vi "Lab13_ThingWorx_WriteToCloud_Bennett.vi"() -> ()   [LabVIEW 2016]
uses:
  <vilib>/National Instruments/IoT Education Toolkit Beta/TW API/TW_SetPropertyValue_Int_Public.vi
  <vilib>/National Instruments/IoT Education Toolkit Beta/TW API/TW_SetPropertyValue_Timestamp_Public.vi
  <vilib>/National Instruments/IoT Education Toolkit Beta/TW API/TW_SetPropertyValue_String_Public.vi
  <vilib>/National Instruments/IoT Education Toolkit Beta/TW API/Properties.lvclass
  <vilib>/National Instruments/IoT Education Toolkit Beta/TW API/Thing.lvclass
panel:
  out "Num of Char":i16=5
  in  "Char":string
  in  "Input String":string
  in  "Input":i32(slide)=5 scale=0.0..10.0
  out "URL":string[](array[string])
  in  "Stop":bool
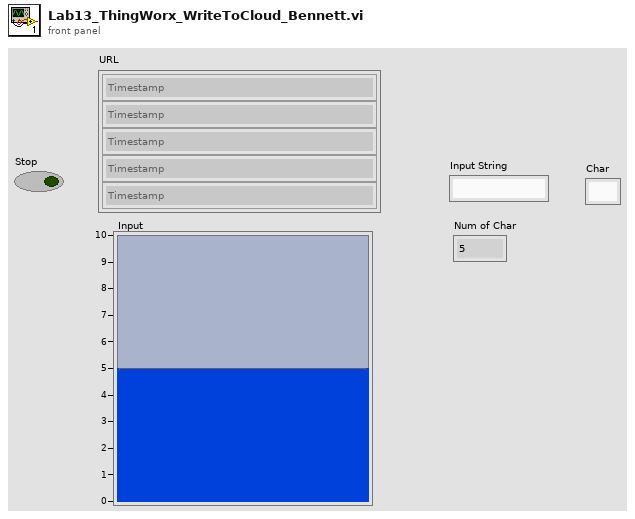
[diagram p1: front panel]
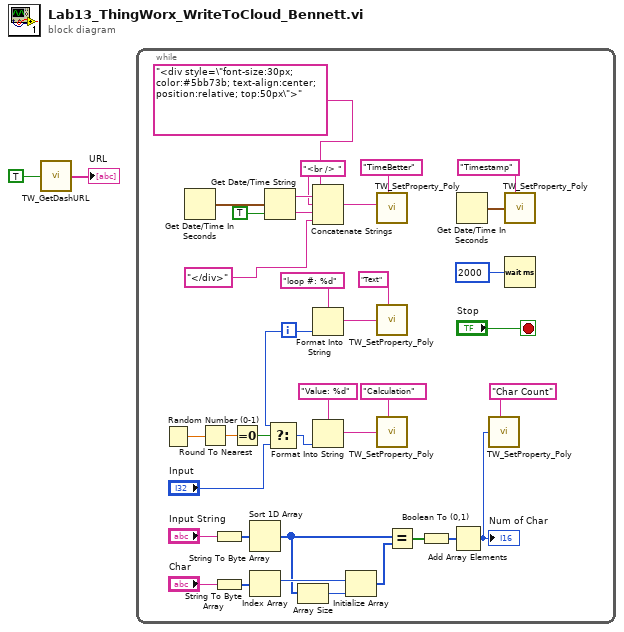
[diagram p0: block diagram]
diagram:
  n1 = call <vilib>:"TW_GetDashURL.vi"("Open Webpage?"=TRUE) -> ("Links"=→"URL":string[])  [unwired: 4 in, 2 out]
  n2 = while {
    i -> [w17]
    stop <- "Stop" stop-if-true
    n3 = Random Number (0-1)() -> (number: 0 to 1=w22:dbl)
    n4 = Get Date/Time In Seconds() -> (seconds since 1Jan1904=w30:timestamp)
    n5 = Round To Nearest(number=w22) -> (nearest integer value=w21:dbl)
    n6 = String To Byte Array(string="Input String") -> (unsigned byte array=w13:u8[])
    n7 = String To Byte Array(string="Char") -> (unsigned byte array=w14:u8[])
    n8 = Equal To 0?(x=w21) -> (x = 0?=w20:bool)
    n9 = Sort 1D Array(array=w13) -> (sorted array=w10:u8[])
    n10 = Index Array(array=w14) -> (element=w12:u8)  [unwired: 1 in]
    n11 = Get Date/Time String(seconds (now)=w30, want seconds? (F)=TRUE) -> (date string=w29:string, time string=w28:string)  [unwired: 1 in]
    n12 = Select(t=w17, s=w20, f="Input") -> (s? t:f=w19:i32)
    n13 = Array Size(array=w10) -> (size(s)=w11:i32)
    n14 = Concatenate Strings("<div style=\"font-size:30px; color:#5bb73b; text-align:center; position:relative; top:50px\">", w29, "<br /> ", w28, "</div>") -> (w26:string)
    n15 = Format Into String(format string="loop #: %d", w17) -> (resulting string=w33:string)  [unwired: 2 in, 1 out]
    n16 = Format Into String(format string="Value: %d", w19) -> (resulting string=w23:string)  [unwired: 2 in, 1 out]
    n17 = Initialize Array(w12, w11) -> (w9:u8[])
    n18 = call-poly <vilib>:"TW_SetProperty_Poly.vi"("Property name"="TimeBetter", "Value"=w26) -> ()  [unwired: 4 in, 2 out]
    n19 = call-poly <vilib>:"TW_SetProperty_Poly.vi"("Property name"="Text", "Value"=w33) -> ()  [unwired: 4 in, 2 out]
    n20 = call-poly <vilib>:"TW_SetProperty_Poly.vi"("Property name"="Calculation", "Value"=w23) -> ()  [unwired: 4 in, 2 out]
    n21 = Equal?(x=w10, y=w9) -> (x = y?=w8:bool[])
    n22 = Boolean To (0,1)(Boolean=w8) -> (0, 1=w7:i16[])
    n23 = Add Array Elements(numeric array=w7) -> (sum=w5:i16)
    "Num of Char" <- w5
    n24 = Get Date/Time In Seconds() -> (seconds since 1Jan1904=w37:timestamp)
    n25 = call-poly <vilib>:"TW_SetProperty_Poly.vi"("Property name"="Char Count", "Value"=w5) -> ()  [unwired: 4 in, 2 out]
    n26 = call-poly <vilib>:"TW_SetProperty_Poly.vi"("Property name"="Timestamp", "time"=w37) -> ()  [unwired: 4 in, 2 out]
    n27 = Wait (ms)(milliseconds to wait=u32 2000) -> ()  [unwired: 1 out]
  }
